vi "ChineseCharacter2Pinyin.vi"(8 "error in (no error)":errorcluster, 11 "Char":string="4lç\u0001") -> (0 "error out":errorcluster, 3 "Pinyin":string)   [LabVIEW 2015]
uses:
  C:/Program Files (x86)/Microsoft Visual Studio International Pack/Simplified Chinese Pin-Yin Conversion Library/ChnCharInfo.dll
  Program Files (x86)/Microsoft Visual Studio International Pack/Simplified Chinese Pin-Yin Conversion Library/ChnCharInfo.dll
panel:
  out "GetBytes":u8[](array[numeric]) format="%.0x"
  out "GetString":string
  out "unicode":u16 format="%.0x"
  out "ASCII":u8[](array[numeric]) format="%.0x"
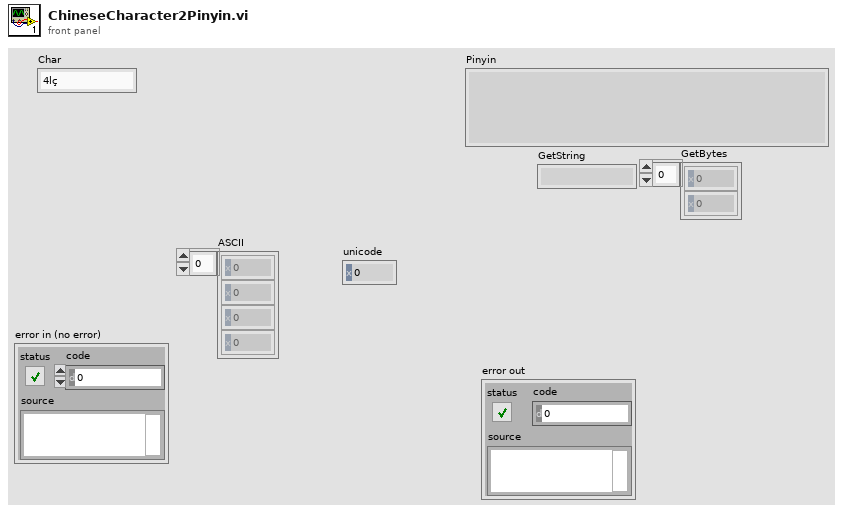
[diagram p1: front panel]
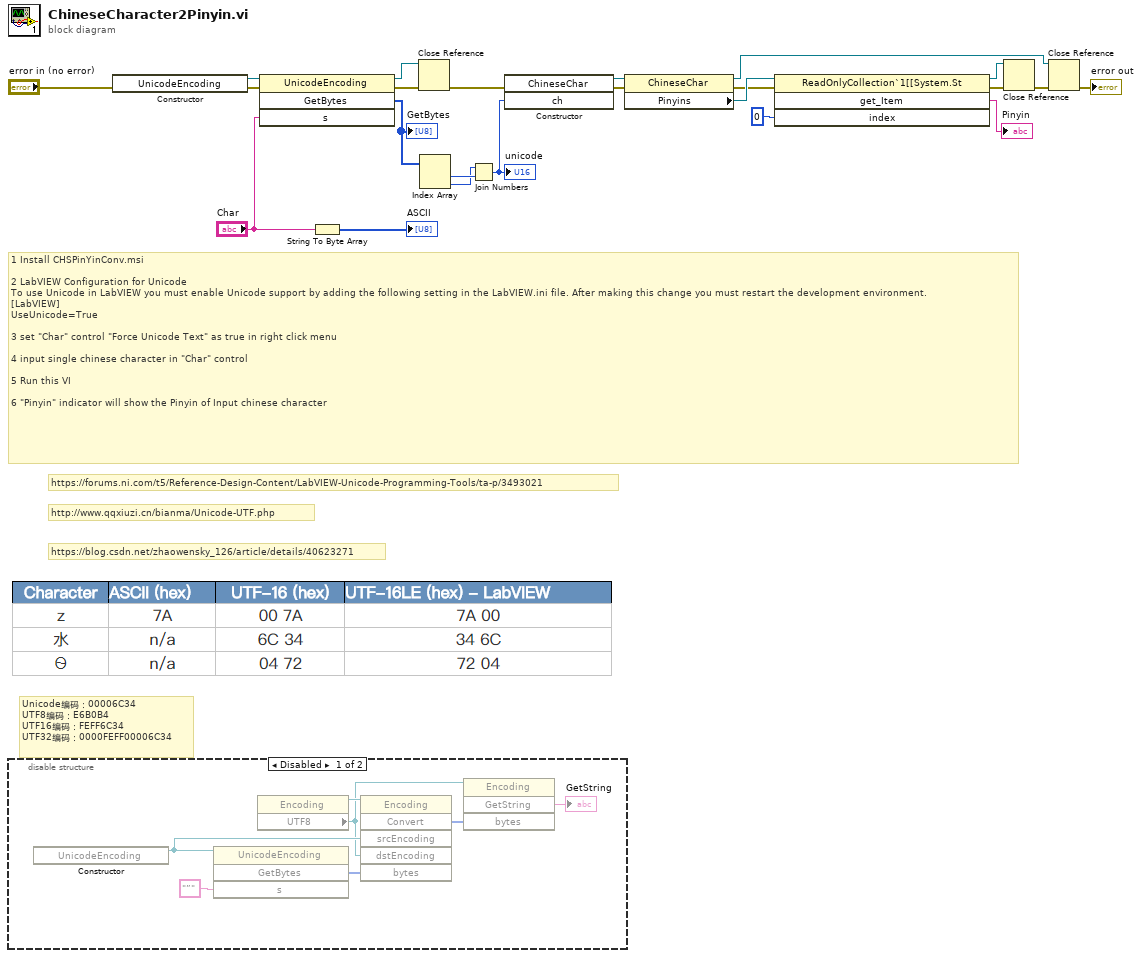
[diagram p0: block diagram]
diagram:
  # "Unicode编码：00006C34\nUTF8编码：E6B0B4\nUTF16编码：FEFF6C34\nUTF32编码：0000FEFF00006C34"
  # "https://blog.csdn.net/zhaowensky_126/article/details/40623271"
  # "http://www.qqxiuzi.cn/bianma/Unicode-UTF.php"
  # "https://forums.ni.com/t5/Reference-Design-Content/LabVIEW-Unicode-Programming-Tools/ta-p/3493021"
  # "1 Install CHSPinYinConv.msi\n\n2 LabVIEW Configuration for Unicode\nTo use Unicode in LabVIEW you must enable Unicode support by adding the following setting in the LabVIEW.ini file. After making this change you must restart the development environment.\n[LabVIEW]\nUseUnicode=True\n\n3 set \"Char\" control \"Force Unicode Text\" as true in right click menu\n\n4 input single chinese character in \"Char\" control \n\n5 Run this VI\n\n6 \"Pinyin\" indicator will show the Pinyin of Input chinese character"
  n1 = disable-structure shown="Disabled" {
    frame Disabled {
      n2 = constructor class="UnicodeEncoding"() -> (reference out=w29:refnum<k24>)  [unwired: 3 in, 2 out]
      n3 = invoke class="UnicodeEncoding" method="GetBytes"(reference=w29, "s"="ˮ") -> ("GetBytes"=w28:u8[])  [unwired: 2 in, 3 out]
      n4 = property class="Encoding"() -> (reference out=w27:refnum<k24>, "UTF8"=w24:refnum<k24>)  [unwired: 2 in, 1 out]
      n5 = invoke class="Encoding" method="Convert"(reference=w27, "srcEncoding"=w29, "dstEncoding"=w24, "bytes"=w28) -> ("Convert"=w26:u8[])  [unwired: 2 in, 5 out]
      n6 = invoke class="Encoding" method="GetString"(reference=w24, "bytes"=w26) -> ("GetString"=→"GetString":string)  [unwired: 2 in, 3 out]
    }
    frame Enabled {
    }
  }
  n7 = constructor class="UnicodeEncoding"(error in="error in (no error)") -> (reference out=w10:refnum<k24>, error out=w5:errorcluster)  [unwired: 2 in, 1 out]
  n8 = invoke class="UnicodeEncoding" method="GetBytes"(reference=w10, error in=w5, "s"="Char") -> (reference out=w4:refnum<k24>, error out=w3:errorcluster, "GetBytes"=w8:u8[])  [unwired: 1 in, 1 out]
  "GetBytes" <- w8
  n9 = String To Byte Array(string="Char") -> (unsigned byte array=→"ASCII":u8[])
  n10 = Close Reference(reference=w4, error in (no error)=w3) -> (error out=w2:errorcluster)
  n11 = Index Array(array=w8) -> (element #1=w7:u8, element #2=w6:u8)  [unwired: 2 in]
  n12 = Join Numbers(hi=w6, lo=w7) -> ((hi.lo)=w18:u16)
  "unicode" <- w18
  n13 = constructor class="ChineseChar"(error in=w2, "ch"=w18) -> (reference out=w20:refnum<k24>, error out=w17:errorcluster)  [unwired: 2 in, 2 out]
  n14 = property class="ChineseChar"(reference=w20, error in=w17) -> (reference out=w12:refnum<k24>, error out=w16:errorcluster, "Pinyins"=w23:refnum<k24>)
  n15 = invoke class="ReadOnlyCollection`1[[System.St" method="get_Item"(reference=w23, error in=w16, "index"=0) -> (reference out=w15:refnum<k24>, error out=w14:errorcluster, "get_Item"=→"Pinyin":string)  [unwired: 1 in, 1 out]
  n16 = Close Reference(reference=w15, error in (no error)=w14) -> (error out=w13:errorcluster)
  n17 = Close Reference(reference=w12, error in (no error)=w13) -> (error out=→"error out":errorcluster)
